vi "Open_Monitor_Config.vi"   [LabVIEW 2016]
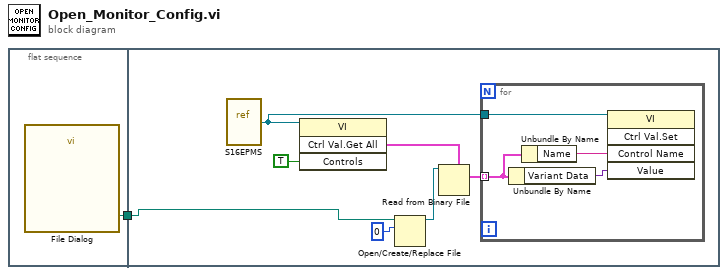
[diagram p0: block diagram]
diagram:
  n1 = flat-sequence {
    tunnel: [w2] -> w1
    tunnel: w1 -> [w3]
    frame #0 {
      n2 = call "File Dialog"() -> ("selected path"=w2:path)  [unwired: 12 in, 3 out]
    }
    frame #1 {
      n3 = vi-ref "S16EPMS.vi"() -> (w8:refnum<vi>)
      n4 = invoke class="VI" method="Ctrl Val.Get All"(reference=w8, "Controls"=TRUE) -> ("Get All Control Values Variant"=w4:cluster{"Name":string, "Variant Data":variant}[])  [unwired: 2 in, 3 out]
      n5 = Open/Create/Replace File(file path (use dialog)=w3, operation (0:open)=0) -> (refnum out=w6:refnum<file>)  [unwired: 4 in, 2 out]
      n6 = Read from Binary File(5:w4, 11:w6) -> (2:w5:cluster{"Name":string, "Variant Data":variant}[])  [unwired: 4 in, 3 out]
      n7 = for {
        tunnel: w8 -> [w13]
        tunnel: w5 -> [w10] mode=indexing
        n8 = Unbundle By Name(w10) -> ("Variant Data"=w11:variant)
        n9 = Unbundle By Name(w10) -> ("Name"=w12:string)
        n10 = invoke class="VI" method="Ctrl Val.Set"(reference=w13, "Control Name"=w12, "Value"=w11) -> ()  [unwired: 2 in, 5 out]
      }
    }
  }
